vi "timming_array_to_digital_waveform.vi"(3 "timing array":dbl[](array[numeric])) -> (0 "Digital Waveform Graph":digitalwaveform(graph))   [LabVIEW 2011]
uses:
  <vilib>/Waveform/DWDTOps.llb/DWDT Boolean Array to Digital.vi
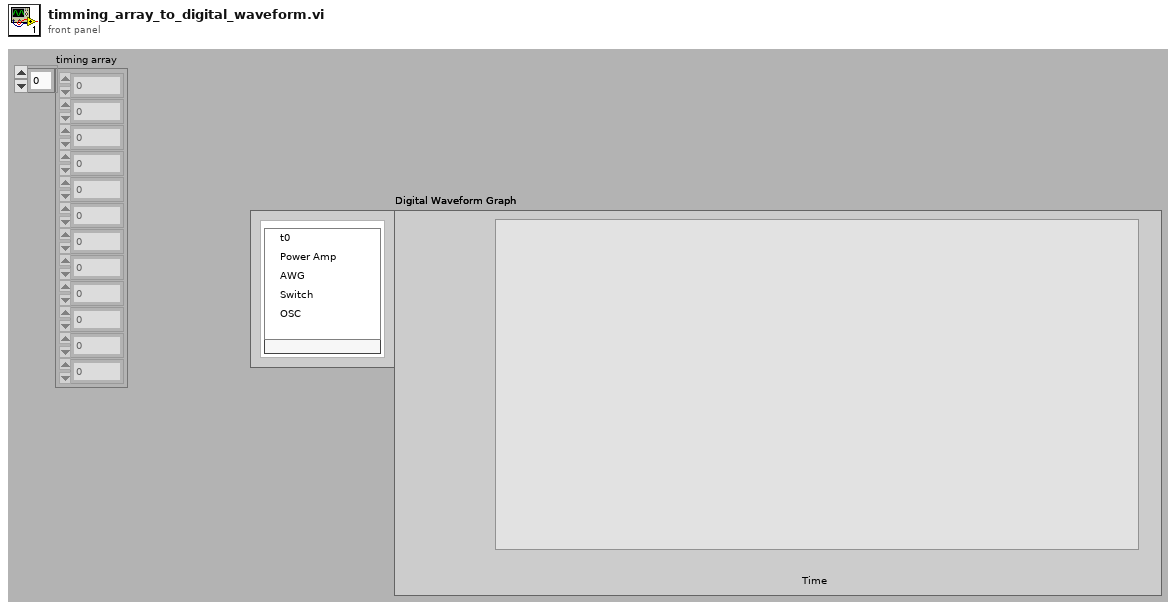
[diagram p1: front panel]
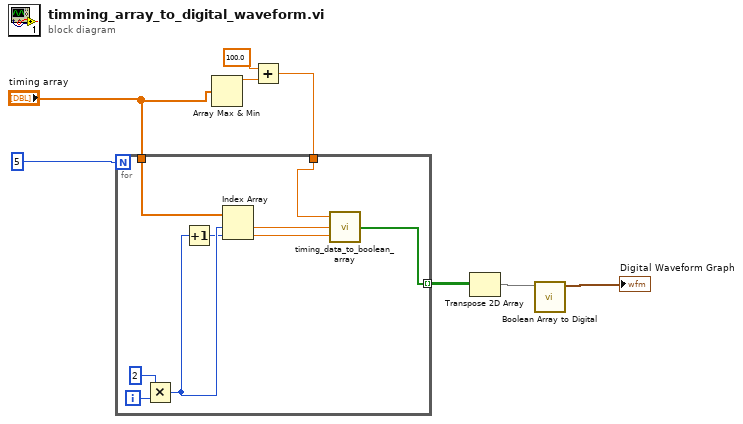
[diagram p0: block diagram]
diagram:
  n1 = Array Max & Min(array="timing array") -> (max value=w3:dbl)  [unwired: 3 out]
  n2 = Add(x=100.0, y=w3) -> (x+y=w1:dbl)
  n3 = for {
    N: 5 -> [_]
    tunnel: [w15] -> w7 mode=indexing
    tunnel: w1 -> [w14]
    tunnel: "timing array" -> [w12]
    i -> [w17]
    n4 = Multiply(x=2, y=w17) -> (x*y=w13:i32)
    n5 = Increment(x=w13) -> (x+1=w11:i32)
    n6 = Index Array(array=w12, index #1=w13, index #2=w11) -> (element #1=w10:dbl, element #2=w9:dbl)
    n7 = call "timing_data_to_boolean_array.vi"("end time [us]"=w9, "start time [us]"=w10, "overall length [us]"=w14) -> ("boolean timing array"=w15:bool[])  [unwired: 1 in]
  }
  n8 = Transpose 2D Array(2D array=w7) -> (transposed array=w6:bool[][])
  n9 = call-poly <vilib>:"Boolean Array to Digital.vi"("boolean array"=w6) -> ("digital waveform"=→"Digital Waveform Graph":digitalwaveform)  [unwired: 9 in, 1 out]
